vi "Write Value Class.vi"(8 "error in (no error)":errorcluster, 10 "Abs_Type.lvclass":refnum<class "Abs_Type.lvclass">, 11 "abs_Type Leaf in":refnum<class "abs_Type Leaf.lvclass">) -> (0 "error out":errorcluster, 3 "abs_Type Leaf out":refnum<class "abs_Type Leaf.lvclass">)   [LabVIEW 2021, in "BT AbsType.lvlib" / "abs_Type Leaf.lvclass"]
uses:
  abs_Type Leaf.lvclass
  <vilib>/TSA/Abstract Data Classes/Abs_Types/Type/Abs_Type.lvclass
  abs_Type Leaf.lvclass/abs_Type Leaf.ctl
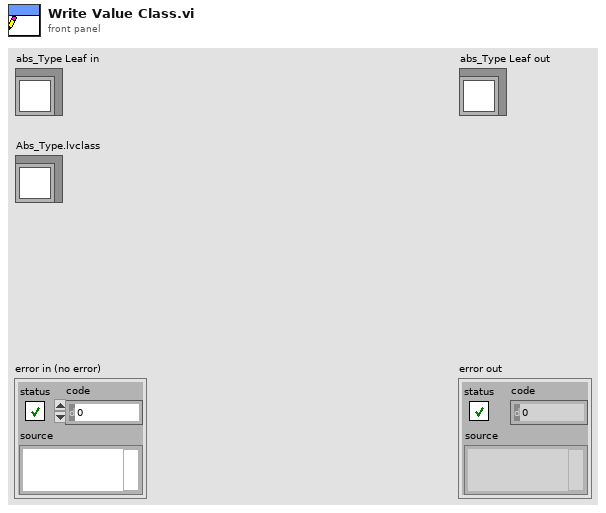
[diagram p1: front panel]
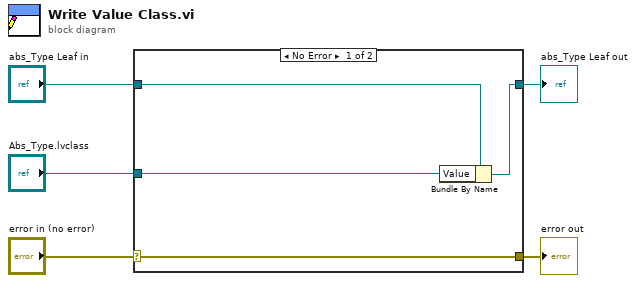
[diagram p0: block diagram]
diagram:
  n1 = case shown="No Error" "error in (no error)" {
    selector: "error in (no error)" -> [w9 w10]
    tunnel: [w9 w10] -> w4
    tunnel: [w7 w11] -> w2
    tunnel: "abs_Type Leaf in" -> [w8 w11]
    tunnel: "Abs_Type.lvclass" -> [w6 _]
    frame No Error {
      n2 = Bundle By Name(cluster=w8, "Value"=w6) -> (w7:refnum<class "abs_Type Leaf.lvclass">)
    }
    frame Error {
    }
  }
  "error out" <- w4
  "abs_Type Leaf out" <- w2
